vi "(SubVI) Set Scanrate and Pull_PI_YCC.vi"(0 "toward+ ?\nT=+, F=-":bool, 2 "axis":u32=1, 3 "scan rate  (um/s)":dbl=2.0 format="%.3f", 5 "range  (um)":dbl=2.0 min=0.0 max=100.0 step=0.5 format="%.3f") -> (1 "Start From  (um)":dbl min=0.0 max=100.0 step=0.5 format="%.3f")   [LabVIEW 2014]
panel:
  out "Velocity":dbl[](array[numeric]) format="%.6f"
  out "Waveform Graph":dbl[](graph)
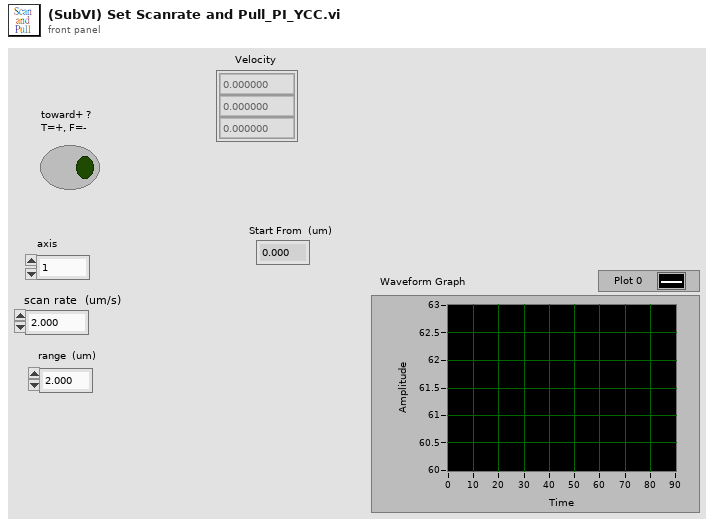
[diagram p1: front panel]
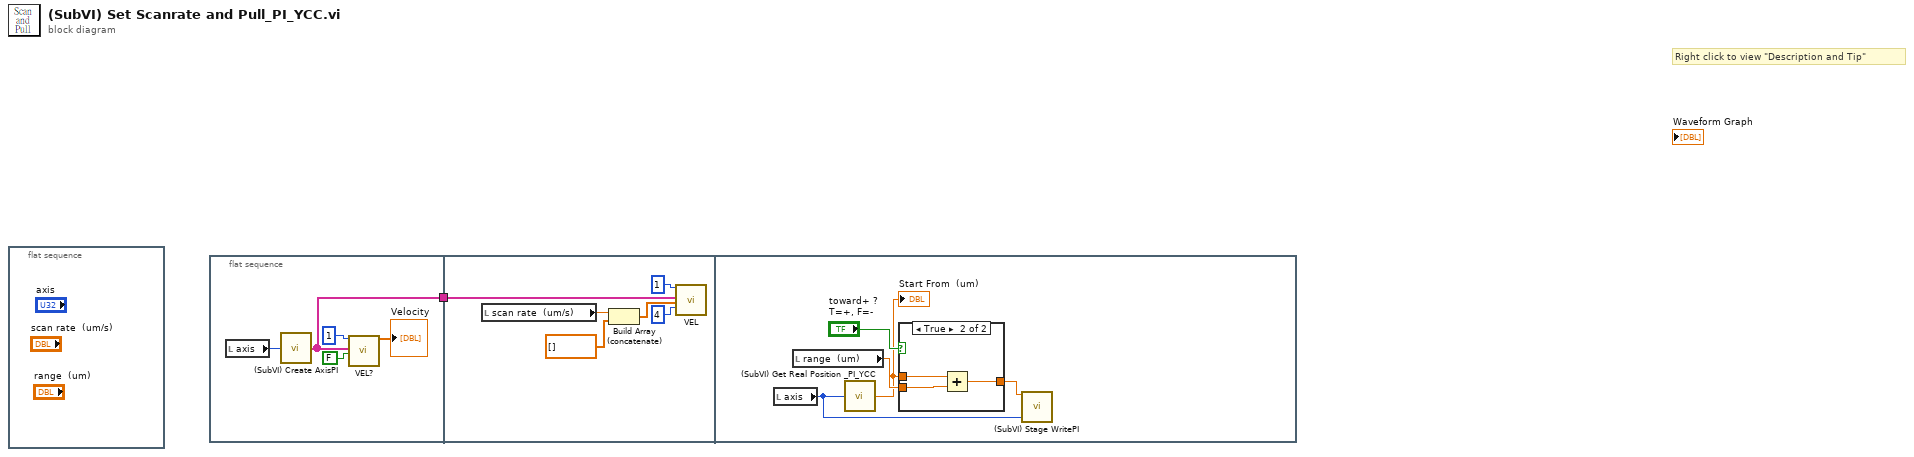
[diagram p0: block diagram]
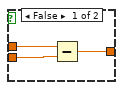
[diagram p2: hidden frame]
diagram:
  # "Right click to view \"Description and Tip\""
  n1 = flat-sequence {
    frame #0 {
    }
  }
  n2 = flat-sequence {
    tunnel: [w3] -> w1
    tunnel: w1 -> [w7]
    frame #0 {
      n3 = local read "axis"() -> (w2:u32)
      n4 = call "(SubVI) Create AxisPI.vi"("axis"=w2) -> ("Array"=w3:string[])  [unwired: 4 in]
      n5 = call "VEL?.vi"("System no."=1, "Axes to query"=w3, "All axes?"=FALSE) -> ("Velocity"=→"Velocity":dbl[])  [unwired: 15 in, 1 out]
    }
    frame #1 {
      n6 = local read "scan rate  (um/s)"() -> (w8:dbl)
      n7 = Build Array (concatenate)(w8, dbl[] []) -> (w10:dbl[])
      n8 = call "VEL.vi"("System no."=1, "Axes to set"=w7, "Velocity values"=w10, "No.of digits"=i16 4) -> ()  [unwired: 14 in, 2 out]
    }
    frame #2 {
      n9 = local read "axis"() -> (w14:u32)
      n10 = local read "range  (um)"() -> (w16:dbl)
      n11 = call "(SubVI) Get Real Position _PI_YCC.vi"("Axis"=w14) -> ("Real Current Commanded position (um)"=w13:dbl)  [unwired: 4 in]
      "Start From  (um)" <- w13
      n12 = case shown="True" "toward+ ?\nT=+, F=-" {
        tunnel: w13 -> [w20 w23]
        tunnel: [w19 w22] -> w15
        tunnel: w16 -> [w18 w21]
        frame False {
          n13 = Subtract(x=w20, y=w18) -> (x-y=w19:dbl)
        }
        frame True {
          n14 = Add(x=w23, y=w21) -> (x+y=w22:dbl)
        }
      }
      n15 = call "(SubVI) Stage WritePI.vi"("axis"=w14, "position"=w15) -> ()  [unwired: 4 in]
    }
  }
